vi "Autodetect Fallback to JSON on Disk.vi"(8 "error in (no error)":errorcluster, 10 "SLSC Module Resource":refnum<k21>, 11 "SLSC Switch Custom Device Ref in":T1 format="%.0x") -> (0 "error out":errorcluster, 2 "Fallback successful?":bool, 3 "SLSC Switch Custom Device Ref out":T1 format="%.0x")   [LabVIEW 2017, in "NI-SWITCH System Explorer.lvlib"]
uses:
  NI-SWITCH System Explorer.lvlib
  <vilib>/NI Veristand/Custom Device API/Custom Device Item Ref.ctl
  <vilib>/Utility/sysdir.llb/System Directory Type.ctl
  Scripting/NI-SWITCH Scripting.lvlib
  <vilib>/NI VeriStand/Custom Device API/Custom Device API.lvlib
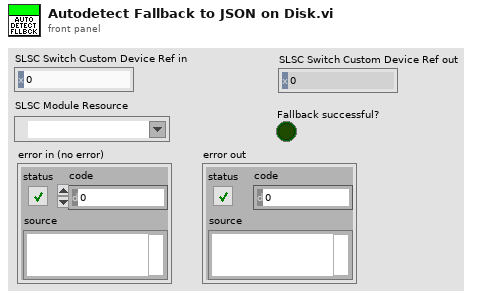
[diagram p1: front panel]
types:
  T1 = typedef "Custom Device API.lvlib/Custom Device Item Ref.ctl" = u64
  T2 = typedef "System Directory Type.ctl" = i32
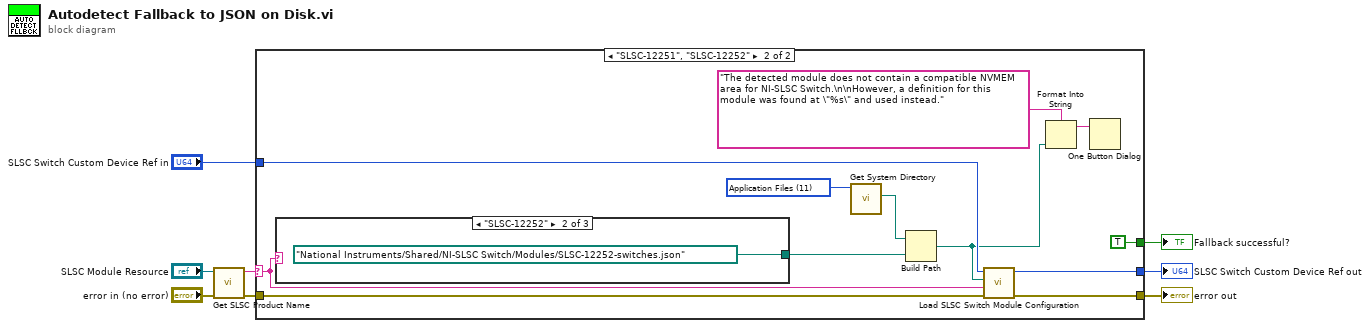
[diagram p0: block diagram]
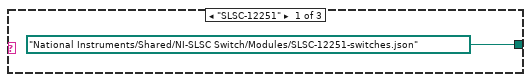
[diagram p3: hidden frame]
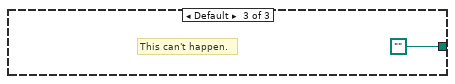
[diagram p4: hidden frame]
diagram:
  n1 = call "Get SLSC Product Name.vi"("error in (no error)"="error in (no error)", "SLSC Module Resource"="SLSC Module Resource") -> ("error out"=w6:errorcluster, "Dev.ProductName"=w5:string)  [unwired: 8 in]
  n2 = case shown="\"SLSC-12251\", \"SLSC-12252\"" w5 {
    selector: w5 -> [_ w21]
    tunnel: w6 -> [w10 w22]
    tunnel: [w10 w18] -> w7
    tunnel: "SLSC Switch Custom Device Ref in" -> [w9 w20]
    tunnel: [w9 w19] -> w2
    tunnel: [_ TRUE] -> w1
    frame Default {
    }
    frame "SLSC-12251", "SLSC-12252" {
      w14 = T2 11 items=["User Home"=0, "User Desktop"=1, "User Documents"=2, "User Application Data"=3, "User Preferences"=4, "User Temporary"=5, "Public Documents"=6, "Public Application Data"=7, "Public Preferences"=8, "Public Cache"=13, "System Core Libraries"=9, "System Installed Libraries"=10, "Application Files"=11, "Boot Volume Root"=12] ("system directory type")
      n3 = case shown="\"SLSC-12252\"" w21 {
        tunnel: [path "National Instruments/Shared/NI-SLSC Switch/Modules/SLSC-12251-switches.json" path "National Instruments/Shared/NI-SLSC Switch/Modules/SLSC-12252-switches.json" path ""] -> w12
        frame "SLSC-12251" {
        }
        frame "SLSC-12252" {
        }
        frame Default {
          # "This can't happen."
        }
      }
      n4 = call <vilib>:"Get System Directory.vi"("system directory type"=w14) -> ("system directory"=w13:path)  [unwired: 10 in]
      n5 = Build Path(base path=w13, name or relative path=w12) -> (appended path=w11:path)
      n6 = call "Load SLSC Switch Module Configuration.vi"("error in"=w22, "product name"=w21, "switches json file"=w11, "slsc switch custom device in"=w20) -> ("error out"=w18:errorcluster, "slsc switch custom device out"=w19:T1)  [unwired: 6 in]
      n7 = Format Into String(format string="The detected module does not contain a compatible NVMEM area for NI-SLSC Switch.\n\nHowever, a definition for this module was found at \"%s\" and used instead.", w11) -> (resulting string=w16:string)  [unwired: 2 in, 1 out]
      n8 = One Button Dialog(message=w16) -> ()  [unwired: 1 in, 1 out]
    }
  }
  "error out" <- w7
  "SLSC Switch Custom Device Ref out" <- w2
  "Fallback successful?" <- w1
